vi "Init.vi"(8 "error in (no error)":errorcluster, 10 "Price":dbl, 11 "Furniture in":refnum<class "Furniture.lvclass">) -> (0 "error out":errorcluster, 3 "Furniture out":refnum<class "Furniture.lvclass">)   [LabVIEW 2019, in "Furniture.lvclass"]
uses:
  Furniture.lvclass
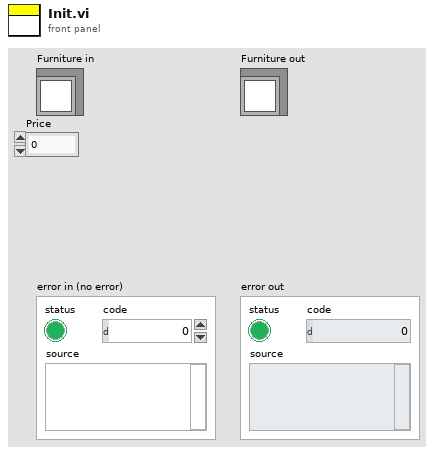
[diagram p1: front panel]
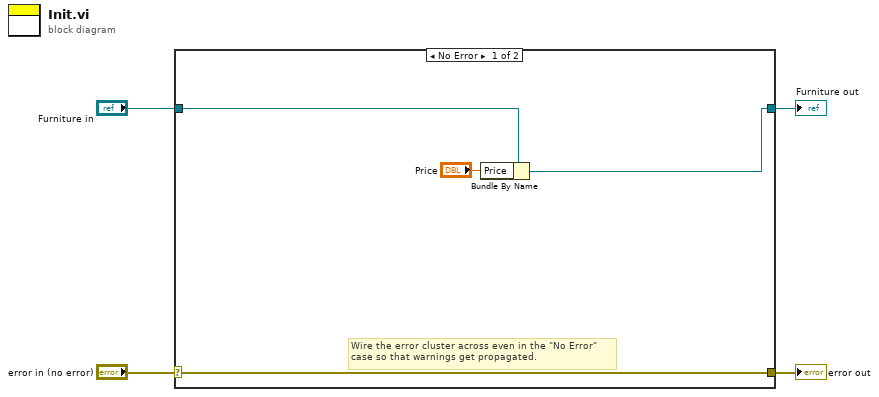
[diagram p0: block diagram]
diagram:
  n1 = case shown="No Error" "error in (no error)" {
    selector: "error in (no error)" -> [w8 w10]
    tunnel: [w8 w10] -> w1
    tunnel: [w6 w9] -> w3
    tunnel: "Furniture in" -> [w7 w9]
    frame No Error {
      # "Wire the error cluster across even in the \"No Error\"\ncase so that warnings get propagated."
      n2 = Bundle By Name(cluster=w7, "Price"="Price") -> (w6:refnum<class "Furniture.lvclass">)
    }
    frame Error {
    }
  }
  "Furniture out" <- w3
  "error out" <- w1
